vi "SA_Random_Solution.vi"(7 "Selection Method":T1, 8 "error in (no error)":errorcluster, 9 "Perturbation Method":T2=enum."NonRedundantSwap", 10 "GA.lvclass":refnum<class "GA.lvclass">, 11 "OSSP_Problem in":refnum<class "OSSP_Problem.lvclass">) -> (0 "error out":errorcluster, 2 "OSSP_Problem out":refnum<class "OSSP_Problem.lvclass">, 3 "GA out":refnum<class "GA.lvclass">)   [LabVIEW 2013]
uses:
  Classes/GA.lvclass
  Classes/OSSP_Problem.lvclass
  Classes/SA_Class/Controls/Perturbation Method.ctl
  Controls/SA Solution Selection Method.ctl
  Classes/SA.lvclass
  SA/Controls/States_SA.ctl
  Classes/OSSP_Problem.lvclass/OSSP_Problem.ctl
  Classes/GA.lvclass/GA.ctl
  Classes/SA_Class/Controls/CoolingScheme.ctl
  Classes/SA.lvclass/SA.ctl
  Classes/SA_Class/Controls/Solution_SA.ctl
  Classes/Graph.lvclass/Graph.ctl
  Classes/GA_Class/Controls/Solution_GA.ctl
  Classes/GanntChart_Class/Operation to Machine Job Tuple.vi
  Classes/GanntChart_Class/Check Other Machines for Schedule Time.vi
  Classes/GanntChart_Class/Schedule Job.vi
  Classes/GanntChart_Class/Find Gaps on Particular Machine.vi
  Classes/GanntChart_Class/Increment Number of Jobs on Machine.vi
  Classes/GanntChart_Class/Find Job On Other Machines.vi
  Remove Duplicates In Array.vi
  Classes/Graph_Class/Create Graph from Solution(Schedule).vi
  Classes/Graph_Class/Find All Paths_DFS.vi
  Classes/Graph_Class/Getters/Read Graph Dictionary.vi
  Classes/Graph_Class/Setters/Write Graph Dictionary.vi
  <userlib>/_OpenG.lib/array/array.llb/Filter 1D Array__ogtk.vi
  <userlib>/_OpenG.lib/array/array.llb/Filter 1D Array (I32)__ogtk.vi
  <userlib>/_OpenG.lib/array/array.llb/Remove Duplicates from 1D Array__ogtk.vi
  <userlib>/_OpenG.lib/array/array.llb/Remove Duplicates from 1D Array (I32)__ogtk.vi
  <userlib>/_OpenG.lib/array/array.llb/Search Array__ogtk.vi
  <userlib>/_OpenG.lib/array/array.llb/Search 1D Array (I32)__ogtk.vi
  <userlib>/_OpenG.lib/array/array.llb/Delete Elements from Array__ogtk.vi
  <userlib>/_OpenG.lib/array/array.llb/Delete Elements from 1D Array (I32)__ogtk.vi
  <userlib>/_OpenG.lib/array/array.llb/Sort Array__ogtk.vi
  <userlib>/_OpenG.lib/array/array.llb/Sort 1D Array (I32)__ogtk.vi
  <userlib>/_OpenG.lib/array/array.llb/Reorder Array2__ogtk.vi
  <userlib>/_OpenG.lib/array/array.llb/Reorder 1D Array2 (I32)__ogtk.vi
  Classes/Graph.lvclass
  Classes/GanntChart.lvclass
panel:
  out "Best Tardiness/Makespan":u16
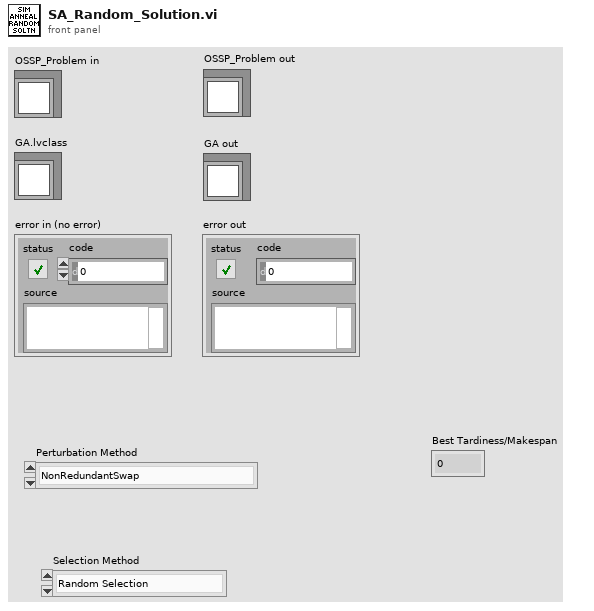
[diagram p1: front panel]
types:
  T1 = typedef "SA Solution Selection Method.ctl" = enum16{"Random Selection", "Tournament Selection"}
  T2 = typedef "SA.lvclass/Perturbation Method.ctl" = enum16{"Simple Swap", "Insert", "NonRedundantSwap", "Job Order Swap", "Machine Order Swap", "Machine&Job Order Swap", "Critical Path Swap"}
  T3 = typedef "States_SA.ctl" = enum16{"Init", "Read Problem", "Sort Problem", "Generate and Evaluate Current Solution", "Perturb Cur Solution and Eval New Solution", "Make Decision", "Keep Track of Best Solution", "Cool", "Output Final Solution", "Stop"}
  T4 = typedef "Solution_GA.ctl" = cluster{"Schedule":u16[], "Fitness":u16, "Fitness Valid?":bool}
  T5 = typedef "Scheduler Type.ctl" = enum16{"Non Delay Scheduler", "GT Active Scheduler", "FIFO Scheduler"}
  T6 = typedef "Objective.ctl" = enum16{"Makespan", "Total Tardiness"}
  T7 = typedef "SA.lvclass/CoolingScheme.ctl" = enum16{"Linear", "Geometric"}
  T8 = typedef "SA.lvclass/Solution_SA.ctl" = cluster{"Schedule":u16[], "Fitness":i16}
  T9 = typedef "GanntChart_Element.ctl" = cluster{"Operation Number":i32, "Job Number":i32, "Start Time":i32, "Procesing Time":u16, "End Time":i32}
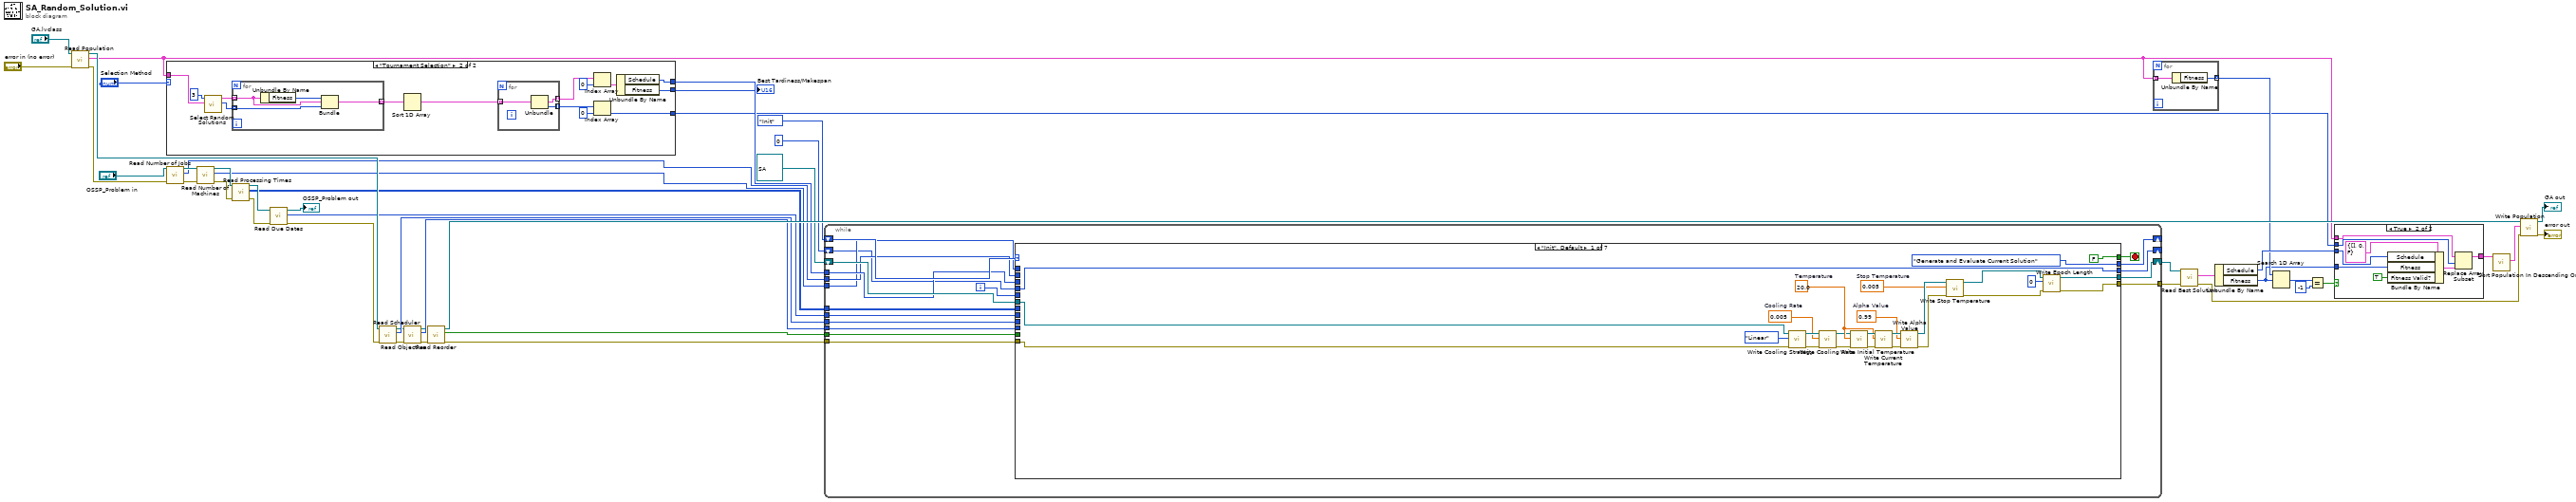
[diagram p0: block diagram]
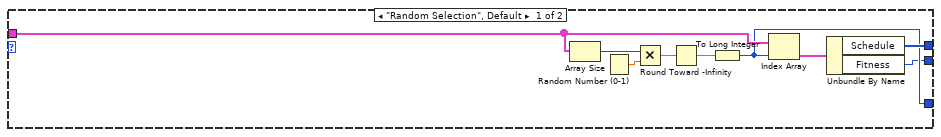
[diagram p2: hidden frame]
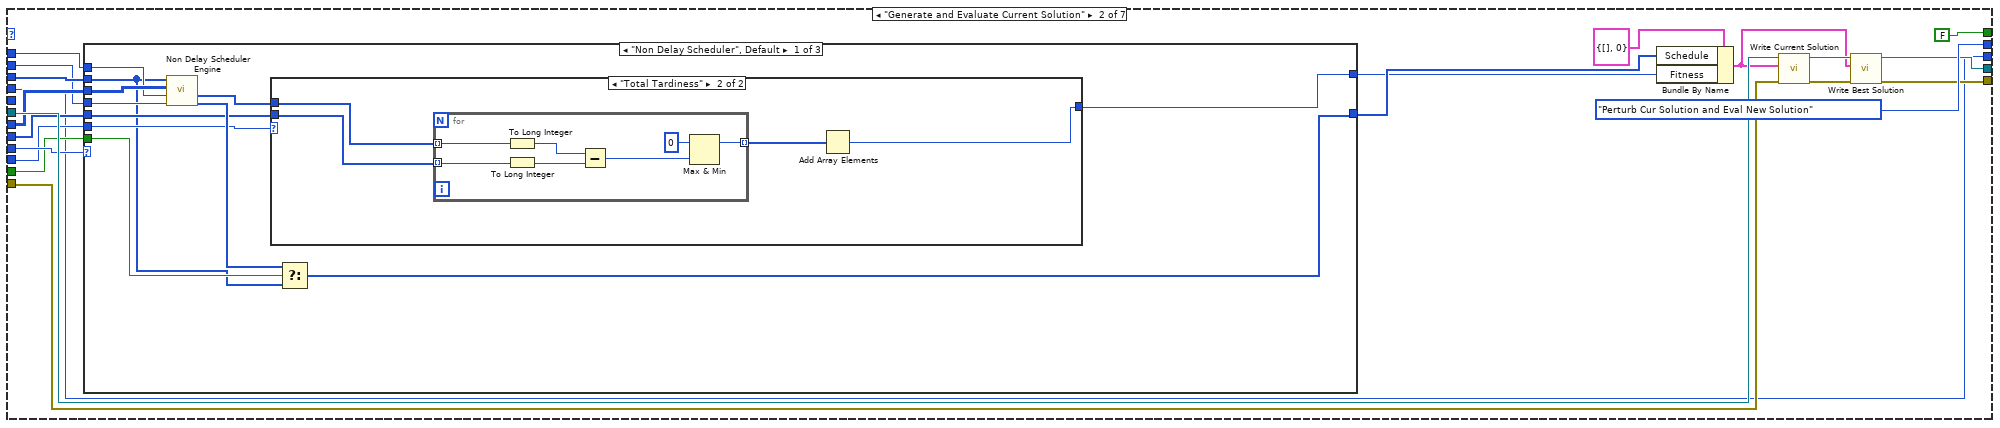
[diagram p4: hidden frame]
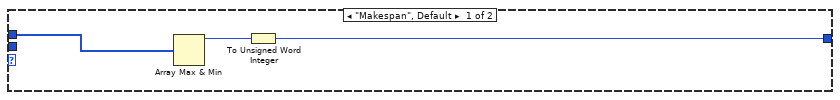
[diagram p5: hidden frame]
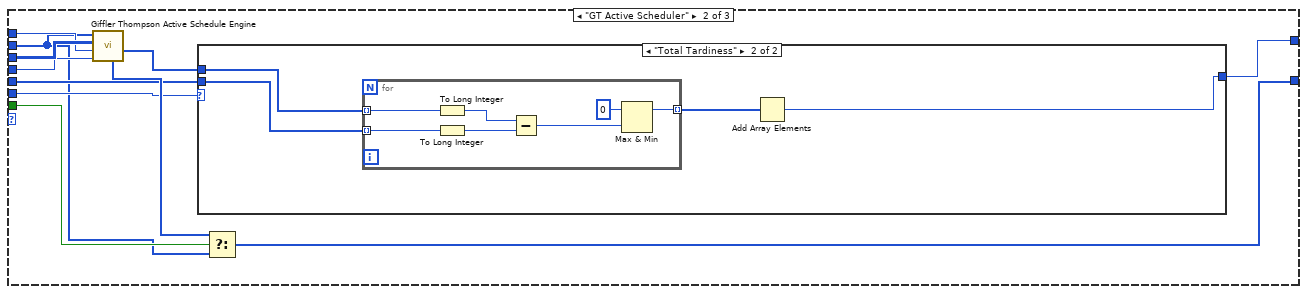
[diagram p6: hidden frame]
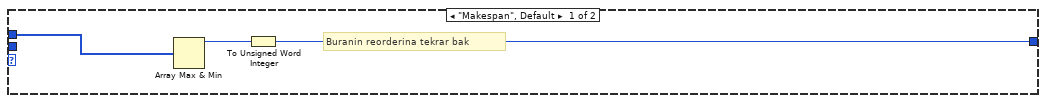
[diagram p7: hidden frame]
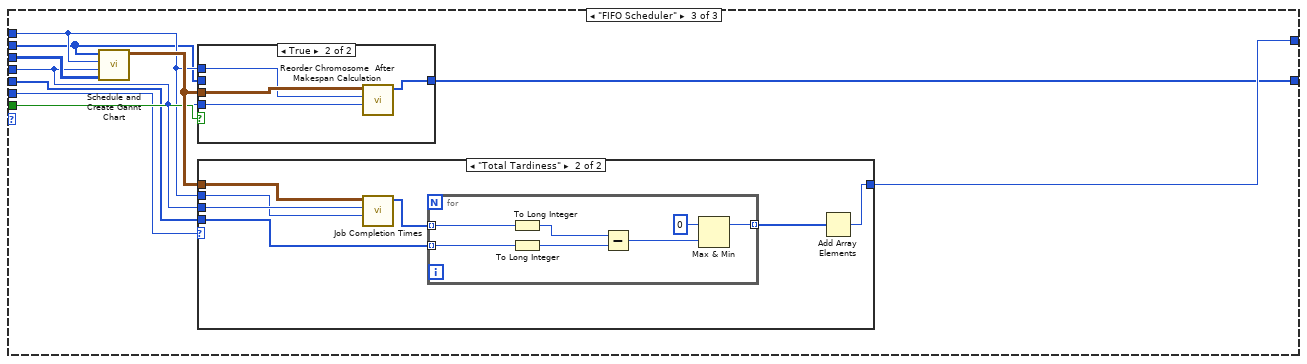
[diagram p8: hidden frame]
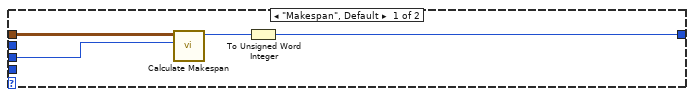
[diagram p10: hidden frame]
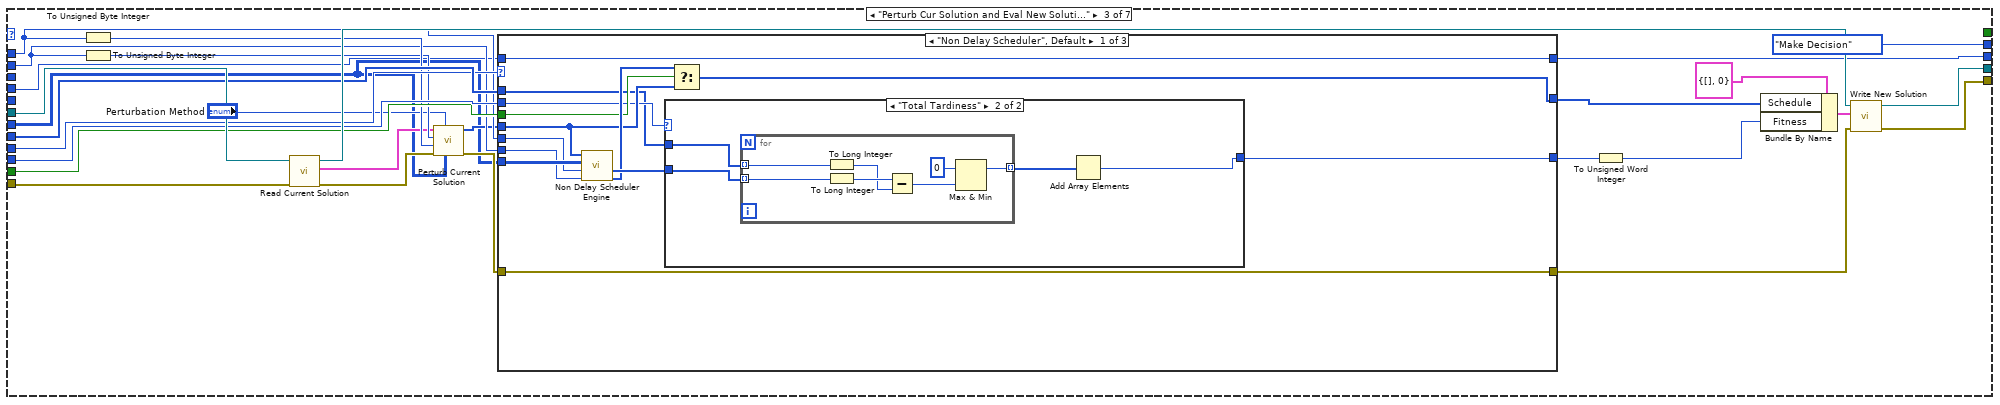
[diagram p11: hidden frame]
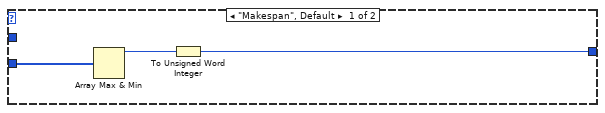
[diagram p12: hidden frame]
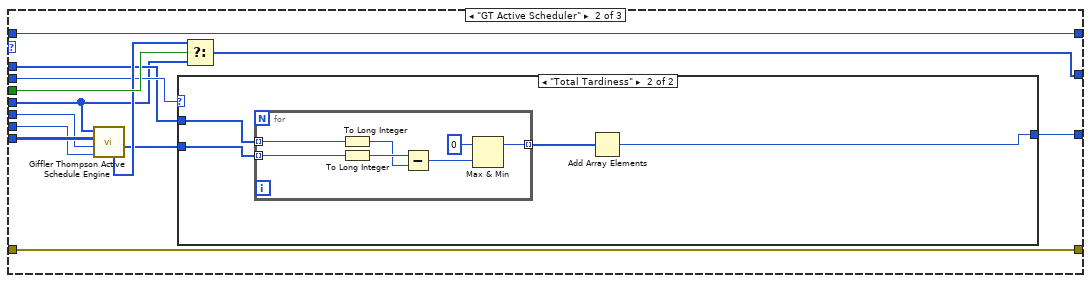
[diagram p13: hidden frame]
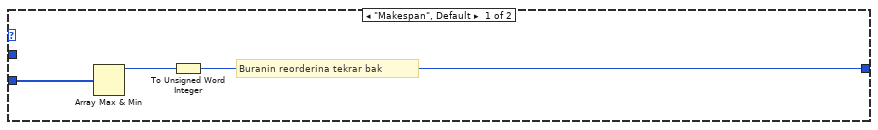
[diagram p14: hidden frame]
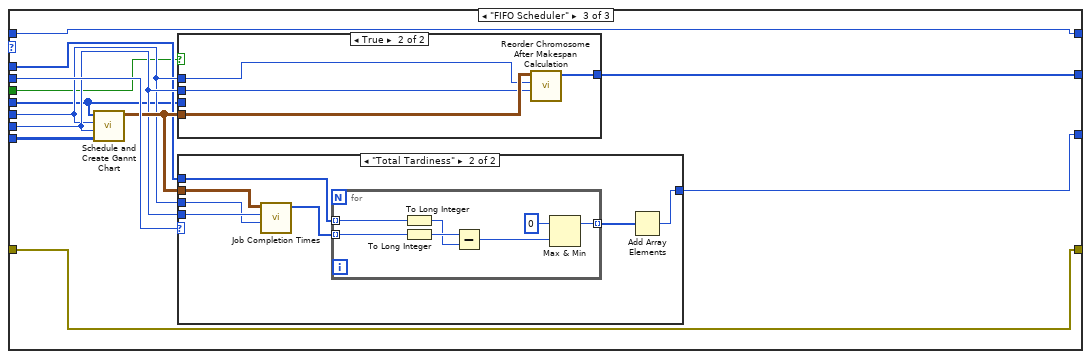
[diagram p15: hidden frame]
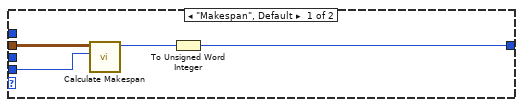
[diagram p17: hidden frame]
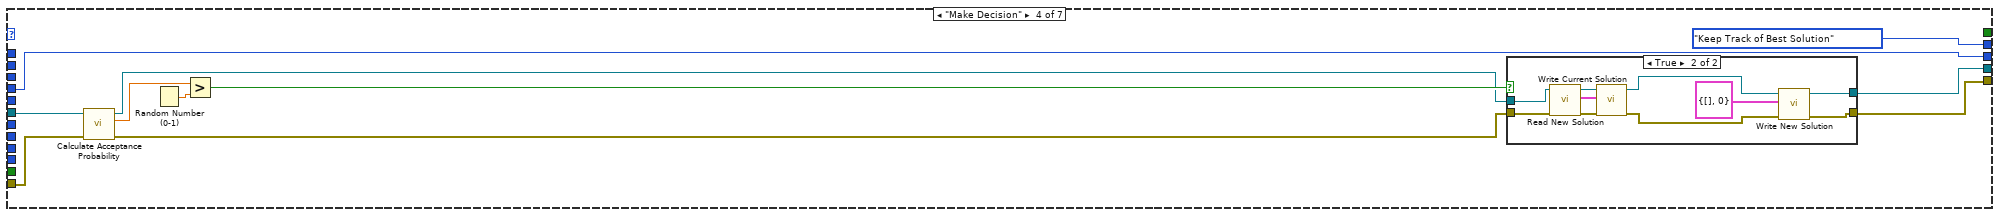
[diagram p18: hidden frame]
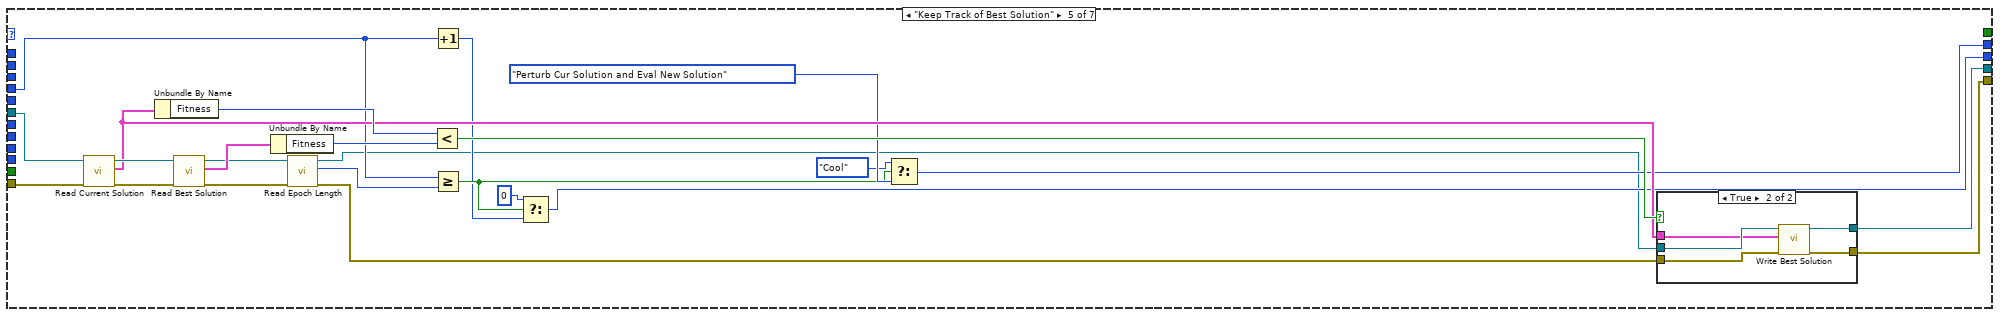
[diagram p20: hidden frame]
diagram:
  n1 = call-dynamic "Read Population.vi"("error in (no error)"="error in (no error)", "GA in"="GA.lvclass") -> ("error out"=w41:errorcluster, "Population"=w5:T4[], "GA out"=w42:refnum<class "GA.lvclass">)  [unwired: 7 in]
  n2 = case shown="\"Tournament Selection\"" "Selection Method" {
    tunnel: w5 -> [w53 w71]
    tunnel: [w51 w63] -> w4
    tunnel: [w50 w58] -> w3
    tunnel: [w49 w62] -> w2
    frame "Random Selection", Default {
      n3 = Array Size(array=w53) -> (size(s)=w56:i32)
      n4 = Random Number (0-1)() -> (number: 0 to 1=w57:dbl)
      n5 = Multiply(x=w56, y=w57) -> (x*y=w55:dbl)
      n6 = Round Toward -Infinity(1:w55) -> (0:w54:dbl)
      n7 = To Long Integer(number=w54) -> (32bit integer=w50:i32)
      n8 = Index Array(array=w53, index=w50) -> (element=w52:T4)
      n9 = Unbundle By Name(w52) -> ("Schedule"=w51:u16[], "Fitness"=w49:u16)
    }
    frame "Tournament Selection" {
      n10 = call "Select Random Solutions.vi"("Population"=w71, "Tournament Size"=3) -> ("Solution Indices"=w61:i32[], "Selected Solutions"=w69:T4[])  [unwired: 8 in]
      n11 = for {
        tunnel: w69 -> [w77] mode=indexing
        tunnel: [w76] -> w68 mode=indexing
        tunnel: w61 -> [w75] mode=indexing
        n12 = Unbundle By Name(w77) -> ("Fitness"=w78:u16)
        n13 = Bundle("Fitness"=w78, "Solution"=w77, w75) -> (w76:cluster{"Fitness":u16, "Solution":T4, i32})  [unwired: 1 in]
      }
      n14 = Sort 1D Array(array=w68) -> (sorted array=w65:cluster{"Fitness":u16, "Solution":T4, i32}[])
      n15 = for {
        tunnel: w65 -> [w74] mode=indexing
        tunnel: [w73] -> w67 mode=indexing
        tunnel: [w72] -> w60 mode=indexing
        n16 = Unbundle(w74) -> ("Solution"=w73:T4, w72:i32)  [unwired: 1 out]
      }
      n17 = Index Array(array=w67, index=0) -> (element=w64:T4)
      n18 = Index Array(array=w60, index=0) -> (element=w58:i32)
      n19 = Unbundle By Name(w64) -> ("Schedule"=w63:u16[], "Fitness"=w62:u16)
    }
  }
  "Best Tardiness/Makespan" <- w2
  n20 = call-dynamic "Read Number of Jobs.vi"("error in (no error)"=w41, "OSSP_Problem in"="OSSP_Problem in") -> ("error out"=w32:errorcluster, "Number of Jobs"=w36:i32, "OSSP_Problem out"=w38:refnum<class "OSSP_Problem.lvclass">)  [unwired: 7 in]
  n21 = call-dynamic "Read Number of Machines.vi"("error in (no error)"=w32, "OSSP_Problem in"=w38) -> ("error out"=w31:errorcluster, "Number of Machines"=w35:i32, "OSSP_Problem out"=w37:refnum<class "OSSP_Problem.lvclass">)  [unwired: 7 in]
  n22 = call-dynamic "Read Processing Times.vi"("error in (no error)"=w31, "OSSP_Problem in"=w37) -> ("error out"=w30:errorcluster, "Processing Times"=w14:u16[][], "OSSP_Problem out"=w29:refnum<class "OSSP_Problem.lvclass">)  [unwired: 7 in]
  n23 = call "Read Due Dates.vi"("error in (no error)"=w30, "OSSP_Problem in"=w29) -> ("error out"=w27:errorcluster, "Due Dates"=w28:u16[], "OSSP_Problem out"=→"OSSP_Problem out":refnum<class "OSSP_Problem.lvclass">)  [unwired: 7 in]
  n24 = call "Read Scheduler.vi"("error in (no error)"=w27, "GA in"=w42) -> ("error out"=w25:errorcluster, "Scheduler"=w26:T5, "GA out"=w24:refnum<class "GA.lvclass">)  [unwired: 7 in]
  n25 = call "Read Objective .vi"("error in (no error)"=w25, "GA in"=w24) -> ("error out"=w22:errorcluster, "Objective"=w23:T6, "GA out"=w19:refnum<class "GA.lvclass">)  [unwired: 7 in]
  n26 = call "Read Reorder.vi"("error in (no error)"=w22, "GA in"=w19) -> ("error out"=w21:errorcluster, "Reorder"=w20:bool, "GA out"=w43:refnum<class "GA.lvclass">)  [unwired: 7 in]
  n27 = while {
    tunnel: w4 -> [w94]
    shift-right: [w89] -> _
    shift-left: States_SA."Init" ("States") -> [w96]
    tunnel: w36 -> [w93]
    tunnel: w35 -> [w92]
    tunnel: w14 -> [w91]
    shift-right: [w90] -> w34
    shift-left: refnum<class "SA.lvclass"> refnum ("SA.lvclass") -> [w95]
    tunnel: [w87] -> w18
    tunnel: w21 -> [w86]
    tunnel: w28 -> [w85]
    tunnel: w26 -> [w84]
    tunnel: w23 -> [w83]
    tunnel: w20 -> [w82]
    shift-right: [w79] -> _
    shift-left: 0 -> [w80]
    i -> [w81]
    stop <- w88 stop-if-true
    n28 = case shown="\"Init\", Default" w96 {
      tunnel: w95 -> [w116 w142 w253 w353 w389 w402 w448]
      tunnel: w94 -> [_ w132 _ _ _ _ _]
      tunnel: w93 -> [_ w129 w236 _ _ _ _]
      tunnel: w92 -> [_ w130 w238 _ _ _ _]
      tunnel: w91 -> [_ w131 w228 _ _ _ _]
      tunnel: [w100 w137 w249 w352 w388 w407 w448] -> w90
      tunnel: [States_SA."Generate and Evaluate Current Solution" ("States") States_SA."Perturb Cur Solution and Eval New Solution" ("States") States_SA."Make Decision" ("States") States_SA."Keep Track of Best Solution" w376 w406 States_SA."Stop"] -> w89
      tunnel: [FALSE FALSE _ _ _ _ TRUE] -> w88
      tunnel: [w98 w123 w246 w345 w379 w404 w446] -> w87
      tunnel: w86 -> [w115 w124 w240 w347 w380 w400 w446]
      tunnel: w85 -> [_ w127 w243 _ _ _ _]
      tunnel: w84 -> [_ w135 w242 _ _ _ _]
      tunnel: w83 -> [_ w134 w241 _ _ _ _]
      tunnel: w82 -> [_ w133 w239 _ _ _ _]
      tunnel: w81 -> [_ _ _ _ _ w403 _]
      tunnel: w80 -> [w102 w122 w227 w344 w375 w397 w445]
      tunnel: [w102 w122 w226 w344 w371 w397 w445] -> w79
      frame "Init", Default {
        w108 = 0.005  # Stop Temperature
        w103 = 0.005  # Cooling Rate
        w120 = 0.99  # Alpha Value
        w111 = 20.0  # Temperature
        n29 = call "Write Cooling Strategy.vi"("error in (no error)"=w115, "Cooling Strategy"=CoolingScheme."Linear", "SA in"=w116) -> ("error out"=w105:errorcluster, "SA out"=w107:refnum<class "SA.lvclass">)  [unwired: 7 in]
        n30 = call "Write Cooling Rate.vi"("error in (no error)"=w105, "Cooling Rate"=w103, "SA in"=w107) -> ("error out"=w104:errorcluster, "SA out"=w106:refnum<class "SA.lvclass">)  [unwired: 7 in]
        n31 = call "Write Initial Temperature.vi"("error in (no error)"=w104, "Initial Temperature"=w111, "SA in"=w106) -> ("error out"=w112:errorcluster, "SA out"=w113:refnum<class "SA.lvclass">)  [unwired: 7 in]
        n32 = call "Write Current Temperature.vi"("error in (no error)"=w112, "Temperature"=w111, "SA in"=w113) -> ("error out"=w117:errorcluster, "SA out"=w121:refnum<class "SA.lvclass">)  [unwired: 7 in]
        n33 = call "Write Alpha Value.vi"("error in (no error)"=w117, "Alpha Value"=w120, "SA in"=w121) -> ("error out"=w109:errorcluster, "SA out"=w110:refnum<class "SA.lvclass">)  [unwired: 7 in]
        n34 = call "Write Stop Temperature.vi"("error in (no error)"=w109, "Stop Temperature"=w108, "SA in"=w110) -> ("error out"=w99:errorcluster, "SA out"=w101:refnum<class "SA.lvclass">)  [unwired: 7 in]
        n35 = call "Write Epoch Length.vi"("error in (no error)"=w99, "Epoch Length"=u8 0, "SA in"=w101) -> ("error out"=w98:errorcluster, "SA out"=w100:refnum<class "SA.lvclass">)  [unwired: 7 in]
      }
      frame "Generate and Evaluate Current Solution" {
        n36 = case shown="\"Non Delay Scheduler\", Default" w135 {
          tunnel: [w149 w174 w202] -> w126
          tunnel: [w150 w175 w200] -> w128
          tunnel: w132 -> [w143 w168 w193]
          tunnel: w133 -> [w151 w178 w199]
          tunnel: w134 -> [w148 w171 w196]
          tunnel: w131 -> [w147 w173 w198]
          tunnel: w130 -> [w146 w170 w195]
          tunnel: w129 -> [w145 w169 w194]
          tunnel: w127 -> [w144 w172 w197]
          frame "Non Delay Scheduler", Default {
            n37 = call "Non Delay Scheduler Engine.vi"("Number of  Jobs"=w145, "Number of Machines"=w146, "Processing Times"=w147, "Schedule"=w143) -> ("Scheduled Jobs Order"=w152:u16[], "Job Completion Times"=w153:u16[])  [unwired: 3 in, 3 out]
            n38 = case shown="\"Total Tardiness\"" w148 {
              tunnel: w153 -> [w156 w160]
              tunnel: [w154 w157] -> w149
              tunnel: w144 -> [_ w159]
              frame "Makespan", Default {
                n39 = Array Max & Min(array=w156) -> (max value=w155:u16)  [unwired: 3 out]
                n40 = To Unsigned Word Integer(number=w155) -> (unsigned 16bit integer=w154:u16)
              }
              frame "Total Tardiness" {
                n41 = for {
                  tunnel: w160 -> [w167] mode=indexing
                  tunnel: w159 -> [w166] mode=indexing
                  tunnel: [w161] -> w158 mode=indexing
                  n42 = To Long Integer(number=w167) -> (32bit integer=w165:i32)
                  n43 = To Long Integer(number=w166) -> (32bit integer=w164:i32)
                  n44 = Subtract(x=w165, y=w164) -> (x-y=w163:i32)
                  n45 = Max & Min(x=0, y=w163) -> (max(x,y)=w161:i32)  [unwired: 1 out]
                }
                n46 = Add Array Elements(numeric array=w158) -> (sum=w157:i32)
              }
            }
            n47 = Select(t=w152, s=w151, f=w143) -> (s? t:f=w150:u16[])
          }
          frame "GT Active Scheduler" {
            n48 = call "Giffler Thompson Active Schedule Engine.vi"("Number of  Jobs"=w169, "Number of Machines"=w170, "Processing Times"=w173, "Schedule In"=w168) -> ("Job Completion Times"=w176:u16[], "Schedule Order"=w177:u16[])  [unwired: 3 in, 3 out]
            n49 = case shown="\"Total Tardiness\"" w171 {
              tunnel: w176 -> [w181 w184]
              tunnel: [w179 w182] -> w174
              tunnel: w172 -> [_ w183]
              frame "Makespan", Default {
                # "Buranin reorderina tekrar bak"
                n50 = Array Max & Min(array=w181) -> (max value=w180:u16)  [unwired: 3 out]
                n51 = To Unsigned Word Integer(number=w180) -> (unsigned 16bit integer=w179:u16)
              }
              frame "Total Tardiness" {
                n52 = for {
                  tunnel: [w188] -> w185 mode=indexing
                  tunnel: w184 -> [w187] mode=indexing
                  tunnel: w183 -> [w186] mode=indexing
                  n53 = To Long Integer(number=w187) -> (32bit integer=w192:i32)
                  n54 = To Long Integer(number=w186) -> (32bit integer=w191:i32)
                  n55 = Subtract(x=w192, y=w191) -> (x-y=w190:i32)
                  n56 = Max & Min(x=0, y=w190) -> (max(x,y)=w188:i32)  [unwired: 1 out]
                }
                n57 = Add Array Elements(numeric array=w185) -> (sum=w182:i32)
              }
            }
            n58 = Select(t=w177, s=w178, f=w168) -> (s? t:f=w175:u16[])
          }
          frame "FIFO Scheduler" {
            n59 = call "Schedule and Create Gannt Chart.vi"("Processing Times (Rows Mach.Cols Jobs)"=w198, "Number of Jobs"=w194, "Number of Machines"=w195, "Schedule"=w193) -> ("Gannt Chart Out"=w201:T9[][])  [unwired: 6 in, 1 out]
            n60 = case shown="True" w199 {
              tunnel: w201 -> [_ w207]
              tunnel: [w203 w206] -> w200
              tunnel: w195 -> [_ w205]
              tunnel: w194 -> [_ w204]
              tunnel: w193 -> [w203 _]
              frame False {
              }
              frame True {
                n61 = call "Reorder Chromosome  After Makespan Calculation.vi"("Number Of  Jobs"=w204, "Number Of Machines"=w205, "Gannt Chart In"=w207) -> ("Reordered Chromosome"=w206:u16[])  [unwired: 8 in]
              }
            }
            n62 = case shown="\"Total Tardiness\"" w196 {
              tunnel: w201 -> [w211 w218]
              tunnel: [w209 w212] -> w202
              tunnel: w197 -> [_ w213]
              tunnel: w194 -> [w208 w217]
              tunnel: w195 -> [_ w216]
              frame "Makespan", Default {
                n63 = call "Calculate Makespan.vi"("Number of Jobs"=w208, "Gannt Chart In"=w211) -> ("Makespan"=w210:i32)  [unwired: 9 in]
                n64 = To Unsigned Word Integer(number=w210) -> (unsigned 16bit integer=w209:u16)
              }
              frame "Total Tardiness" {
                n65 = call "Job Completion Times.vi"("Number Of Machines"=w216, "Number Of Jobs"=w217, "Gannt Chart In"=w218) -> ("Job Completion Times"=w214:u16[])  [unwired: 8 in]
                n66 = for {
                  tunnel: [w221] -> w215 mode=indexing
                  tunnel: w214 -> [w220] mode=indexing
                  tunnel: w213 -> [w219] mode=indexing
                  n67 = To Long Integer(number=w220) -> (32bit integer=w225:i32)
                  n68 = To Long Integer(number=w219) -> (32bit integer=w224:i32)
                  n69 = Subtract(x=w225, y=w224) -> (x-y=w223:i32)
                  n70 = Max & Min(x=0, y=w223) -> (max(x,y)=w221:i32)  [unwired: 1 out]
                }
                n71 = Add Array Elements(numeric array=w215) -> (sum=w212:i32)
              }
            }
          }
        }
        n72 = Bundle By Name(cluster=T8 {"Schedule"=[], "Fitness"=0} ("Solution"), "Schedule"=w128, "Fitness"=w126) -> (w136:T8)
        n73 = call "Write Current Solution.vi"("error in (no error)"=w124, "Solution"=w136, "SA in"=w142) -> ("error out"=w125:errorcluster, "SA out"=w138:refnum<class "SA.lvclass">)  [unwired: 7 in]
        n74 = call "Write Best Solution.vi"("error in (no error)"=w125, "Solution"=w136, "SA in"=w138) -> ("error out"=w123:errorcluster, "SA out"=w137:refnum<class "SA.lvclass">)  [unwired: 7 in]
      }
      frame "Perturb Cur Solution and Eval New Solution" {
        n75 = To Unsigned Byte Integer(number=w238) -> (unsigned 8bit integer=w237:u8)
        n76 = To Unsigned Byte Integer(number=w236) -> (unsigned 8bit integer=w235:u8)
        n77 = call "Read Current Solution.vi"("error in (no error)"=w240, "SA in"=w253) -> ("error out"=w233:errorcluster, "Solution"=w229:T8, "SA out"=w252:refnum<class "SA.lvclass">)  [unwired: 7 in]
        n78 = call "Perturb Current Solution.vi"("Processing Times (Rows Machine, Columns Jobs)"=w228, "Perturbation Method"="Perturbation Method", "error in (no error)"=w233, "Number of Machines"=w237, "Number of Jobs"=w235, "Solution"=w229) -> ("error out"=w232:errorcluster, "Perturbed Schedule"=w230:u16[])  [unwired: 4 in]
        n79 = case shown="\"Non Delay Scheduler\", Default" w242 {
          tunnel: w230 -> [w260 w285 w310]
          tunnel: w238 -> [w262 w287 w313]
          tunnel: w236 -> [w263 w289 w315]
          tunnel: w228 -> [w264 w293 w319]
          tunnel: [w256 w283 w318] -> w245
          tunnel: w241 -> [w258 w288 w317]
          tunnel: [w259 w284 w314] -> w244
          tunnel: w243 -> [w257 w286 w312]
          tunnel: w239 -> [w261 w292 w311]
          tunnel: [w255 w282 w309] -> w231
          tunnel: w232 -> [w255 w282 w309]
          tunnel: w227 -> [w254 w281 w308]
          tunnel: [w254 w281 w308] -> w226
          frame "Non Delay Scheduler", Default {
            n80 = call "Non Delay Scheduler Engine.vi"("Number of  Jobs"=w263, "Number of Machines"=w262, "Processing Times"=w264, "Schedule"=w260) -> ("Scheduled Jobs Order"=w265:u16[], "Job Completion Times"=w266:u16[])  [unwired: 3 in, 3 out]
            n81 = case shown="\"Total Tardiness\"" w258 {
              tunnel: w266 -> [w269 w272]
              tunnel: [w267 w270] -> w256
              tunnel: w257 -> [_ w271]
              frame "Makespan", Default {
                n82 = Array Max & Min(array=w269) -> (max value=w268:u16)  [unwired: 3 out]
                n83 = To Unsigned Word Integer(number=w268) -> (unsigned 16bit integer=w267:u16)
              }
              frame "Total Tardiness" {
                n84 = for {
                  tunnel: w272 -> [w280] mode=indexing
                  tunnel: w271 -> [w279] mode=indexing
                  tunnel: [w274] -> w273 mode=indexing
                  n85 = To Long Integer(number=w279) -> (32bit integer=w277:i32)
                  n86 = To Long Integer(number=w280) -> (32bit integer=w278:i32)
                  n87 = Subtract(x=w278, y=w277) -> (x-y=w276:i32)
                  n88 = Max & Min(x=0, y=w276) -> (max(x,y)=w274:i32)  [unwired: 1 out]
                }
                n89 = Add Array Elements(numeric array=w273) -> (sum=w270:i32)
              }
            }
            n90 = Select(t=w265, s=w261, f=w260) -> (s? t:f=w259:u16[])
          }
          frame "GT Active Scheduler" {
            n91 = call "Giffler Thompson Active Schedule Engine.vi"("Number of  Jobs"=w289, "Number of Machines"=w287, "Processing Times"=w293, "Schedule In"=w285) -> ("Job Completion Times"=w290:u16[], "Schedule Order"=w291:u16[])  [unwired: 3 in, 3 out]
            n92 = case shown="\"Total Tardiness\"" w288 {
              tunnel: w290 -> [w296 w299]
              tunnel: [w294 w297] -> w283
              tunnel: w286 -> [_ w298]
              frame "Makespan", Default {
                # "Buranin reorderina tekrar bak"
                n93 = Array Max & Min(array=w296) -> (max value=w295:u16)  [unwired: 3 out]
                n94 = To Unsigned Word Integer(number=w295) -> (unsigned 16bit integer=w294:u16)
              }
              frame "Total Tardiness" {
                n95 = for {
                  tunnel: [w303] -> w300 mode=indexing
                  tunnel: w299 -> [w302] mode=indexing
                  tunnel: w298 -> [w301] mode=indexing
                  n96 = To Long Integer(number=w301) -> (32bit integer=w306:i32)
                  n97 = To Long Integer(number=w302) -> (32bit integer=w307:i32)
                  n98 = Subtract(x=w307, y=w306) -> (x-y=w305:i32)
                  n99 = Max & Min(x=0, y=w305) -> (max(x,y)=w303:i32)  [unwired: 1 out]
                }
                n100 = Add Array Elements(numeric array=w300) -> (sum=w297:i32)
              }
            }
            n101 = Select(t=w291, s=w292, f=w285) -> (s? t:f=w284:u16[])
          }
          frame "FIFO Scheduler" {
            n102 = call "Schedule and Create Gannt Chart.vi"("Processing Times (Rows Mach.Cols Jobs)"=w319, "Number of Jobs"=w315, "Number of Machines"=w313, "Schedule"=w310) -> ("Gannt Chart Out"=w316:T9[][])  [unwired: 6 in, 1 out]
            n103 = case shown="True" w311 {
              tunnel: w316 -> [_ w324]
              tunnel: w313 -> [_ w323]
              tunnel: w315 -> [_ w322]
              tunnel: [w320 w321] -> w314
              tunnel: w310 -> [w320 _]
              frame False {
              }
              frame True {
                n104 = call "Reorder Chromosome  After Makespan Calculation.vi"("Number Of  Jobs"=w322, "Number Of Machines"=w323, "Gannt Chart In"=w324) -> ("Reordered Chromosome"=w321:u16[])  [unwired: 8 in]
              }
            }
            n105 = case shown="\"Total Tardiness\"" w317 {
              tunnel: w316 -> [w328 w335]
              tunnel: [w325 w329] -> w318
              tunnel: w315 -> [w327 w334]
              tunnel: w313 -> [_ w333]
              tunnel: w312 -> [_ w330]
              frame "Makespan", Default {
                n106 = call "Calculate Makespan.vi"("Number of Jobs"=w327, "Gannt Chart In"=w328) -> ("Makespan"=w326:i32)  [unwired: 9 in]
                n107 = To Unsigned Word Integer(number=w326) -> (unsigned 16bit integer=w325:u16)
              }
              frame "Total Tardiness" {
                n108 = call "Job Completion Times.vi"("Number Of Machines"=w333, "Number Of Jobs"=w334, "Gannt Chart In"=w335) -> ("Job Completion Times"=w331:u16[])  [unwired: 8 in]
                n109 = for {
                  tunnel: [w338] -> w332 mode=indexing
                  tunnel: w331 -> [w337] mode=indexing
                  tunnel: w330 -> [w336] mode=indexing
                  n110 = To Long Integer(number=w336) -> (32bit integer=w341:i32)
                  n111 = To Long Integer(number=w337) -> (32bit integer=w342:i32)
                  n112 = Subtract(x=w342, y=w341) -> (x-y=w340:i32)
                  n113 = Max & Min(x=0, y=w340) -> (max(x,y)=w338:i32)  [unwired: 1 out]
                }
                n114 = Add Array Elements(numeric array=w332) -> (sum=w329:i32)
              }
            }
          }
        }
        n115 = To Unsigned Word Integer(number=w245) -> (unsigned 16bit integer=w247:u16)
        n116 = Bundle By Name(cluster=T8 {"Schedule"=[], "Fitness"=0} ("Solution"), "Schedule"=w244, "Fitness"=w247) -> (w250:T8)
        n117 = call "Write New Solution.vi"("error in (no error)"=w231, "Solution"=w250, "SA in"=w252) -> ("error out"=w246:errorcluster, "SA out"=w249:refnum<class "SA.lvclass">)  [unwired: 7 in]
      }
      frame "Make Decision" {
        n118 = call "Calculate Acceptance Probability.vi"("error in (no error)"=w347, "SA in"=w353) -> ("error out"=w346:errorcluster, "Acceptance Probability"=w351:dbl, "SA out"=w348:refnum<class "SA.lvclass">)  [unwired: 7 in]
        n119 = Random Number (0-1)() -> (number: 0 to 1=w350:dbl)
        n120 = Greater?(x=w351, y=w350) -> (0:w349:bool)
        n121 = case shown="True" w349 {
          tunnel: w348 -> [w355 w365]
          tunnel: [w355 w359] -> w352
          tunnel: w346 -> [w354 w358]
          tunnel: [w354 w357] -> w345
          frame False {
          }
          frame True {
            n122 = call "Read New Solution.vi"("error in (no error)"=w358, "SA in"=w365) -> ("error out"=w364:errorcluster, "Solution"=w362:T8, "SA out"=w363:refnum<class "SA.lvclass">)  [unwired: 7 in]
            n123 = call "Write Current Solution.vi"("error in (no error)"=w364, "Solution"=w362, "SA in"=w363) -> ("error out"=w360:errorcluster, "SA out"=w361:refnum<class "SA.lvclass">)  [unwired: 7 in]
            n124 = call "Write New Solution.vi"("error in (no error)"=w360, "Solution"=T8 {"Schedule"=[], "Fitness"=0}, "SA in"=w361) -> ("error out"=w357:errorcluster, "SA out"=w359:refnum<class "SA.lvclass">)  [unwired: 7 in]
          }
        }
      }
      frame "Keep Track of Best Solution" {
        n125 = call "Read Current Solution.vi"("error in (no error)"=w380, "SA in"=w389) -> ("error out"=w381:errorcluster, "Solution"=w382:T8, "SA out"=w387:refnum<class "SA.lvclass">)  [unwired: 7 in]
        n126 = Unbundle By Name(w382) -> ("Fitness"=w386:i16)
        n127 = call "Read Best Solution.vi"("error in (no error)"=w381, "SA in"=w387) -> ("error out"=w367:errorcluster, "Solution"=w385:T8, "SA out"=w370:refnum<class "SA.lvclass">)  [unwired: 7 in]
        n128 = Unbundle By Name(w385) -> ("Fitness"=w384:i16)
        n129 = call "Read Epoch Length.vi"("error in (no error)"=w367, "SA in"=w370) -> ("error out"=w366:errorcluster, "Epoch Length"=w368:u8, "SA out"=w369:refnum<class "SA.lvclass">)  [unwired: 7 in]
        n130 = Less?(x=w386, y=w384) -> (x < y?=w383:bool)
        n131 = Increment(x=w375) -> (x+1=w373:i32)
        n132 = Greater Or Equal?(x=w375, y=w368) -> (x >= y?=w374:bool)
        n133 = Select(t=0, s=w374, f=w373) -> (s? t:f=w371:i32)
        n134 = Select(t=States_SA."Cool", s=w374, f=States_SA."Perturb Cur Solution and Eval New Solution") -> (s? t:f=w376:T3)
        n135 = case shown="True" w383 {
          tunnel: w369 -> [w391 w396]
          tunnel: [w391 w395] -> w388
          tunnel: w382 -> [_ w394]
          tunnel: w366 -> [w390 w393]
          tunnel: [w390 w392] -> w379
          frame False {
          }
          frame True {
            n136 = call "Write Best Solution.vi"("error in (no error)"=w393, "Solution"=w394, "SA in"=w396) -> ("error out"=w392:errorcluster, "SA out"=w395:refnum<class "SA.lvclass">)  [unwired: 7 in]
          }
        }
      }
      frame "Cool" {
        n137 = call "Read Stop Temperature.vi"("error in (no error)"=w400, "SA in"=w402) -> ("error out"=w399:errorcluster, "Stop Temperature"=w398:dbl, "SA out"=w401:refnum<class "SA.lvclass">)  [unwired: 7 in]
        n138 = call "Read Current Temperature.vi"("error in (no error)"=w399, "SA in"=w401) -> ("error out"=w405:errorcluster, "Temperature"=w408:dbl, "SA out"=w409:refnum<class "SA.lvclass">)  [unwired: 7 in]
        n139 = Less?(x=w408, y=w398) -> (x < y?=w410:bool)
        n140 = case shown="False" w410 {
          tunnel: [States_SA."Perturb Cur Solution and Eval New Solution" ("f") States_SA."Stop"] -> w406
          tunnel: w409 -> [w416 w443]
          tunnel: [w422 w443] -> w407
          tunnel: w408 -> [w418 _]
          tunnel: w405 -> [w414 w442]
          tunnel: [w417 w442] -> w404
          tunnel: w403 -> [w411 _]
          frame False {
            n141 = call "Read Cooling Strategy.vi"("error in (no error)"=w414, "SA in"=w416) -> ("error out"=w413:errorcluster, "Cooling Strategy"=w412:T7, "SA out"=w415:refnum<class "SA.lvclass">)  [unwired: 7 in]
            n142 = case shown="\"Geometric\"" w412 {
              tunnel: w415 -> [w432 w441]
              tunnel: [w431 w433] -> w421
              tunnel: [w430 w436] -> w420
              tunnel: [w426 w439] -> w419
              tunnel: w418 -> [w425 _]
              tunnel: w413 -> [w424 w440]
              tunnel: w411 -> [_ _]
              frame "Linear", Default {
                n143 = call "Read Cooling Rate.vi"("error in (no error)"=w424, "SA in"=w432) -> ("error out"=w430:errorcluster, "Cooling Rate"=w428:dbl, "SA out"=w431:refnum<class "SA.lvclass">)  [unwired: 7 in]
                n144 = Subtract(x=1.0, y=w428) -> (x-y=w427:dbl)
                n145 = Multiply(x=w427, y=w425) -> (x*y=w426:dbl)
              }
              frame "Geometric" {
                n146 = call "Read Alpha Value.vi"("error in (no error)"=w440, "SA in"=w441) -> ("error out"=w437:errorcluster, "Alpha Value"=w435:dbl, "SA out"=w438:refnum<class "SA.lvclass">)  [unwired: 7 in]
                n147 = call "Read Current Temperature.vi"("error in (no error)"=w437, "SA in"=w438) -> ("error out"=w436:errorcluster, "Temperature"=w434:dbl, "SA out"=w433:refnum<class "SA.lvclass">)  [unwired: 7 in]
                n148 = Multiply(x=w435, y=w434) -> (x*y=w439:dbl)
              }
            }
            n149 = call "Write Current Temperature.vi"("error in (no error)"=w420, "Temperature"=w419, "SA in"=w421) -> ("error out"=w417:errorcluster, "SA out"=w422:refnum<class "SA.lvclass">)  [unwired: 7 in]
          }
          frame True {
          }
        }
      }
      frame "Stop" {
      }
    }
  }
  n150 = for {
    tunnel: w5 -> [w451] mode=indexing
    tunnel: [w450] -> w10 mode=indexing
    n151 = Unbundle By Name(w451) -> ("Fitness"=w450:u16)
  }
  n152 = call "Read Best Solution.vi"("error in (no error)"=w18, "SA in"=w34) -> ("error out"=w17:errorcluster, "Solution"=w33:T8)  [unwired: 7 in, 1 out]
  n153 = Unbundle By Name(w33) -> ("Schedule"=w15:u16[], "Fitness"=w9:i16)
  n154 = Search 1D Array(1D array=w10, element=w9) -> (index of element=w12:i32)  [unwired: 1 in]
  n155 = Equal?(x=w12, y=-1) -> (x = y?=w8:bool)
  n156 = case shown="True" w8 {
    tunnel: [w452 w459] -> w7
    tunnel: w15 -> [_ w456]
    tunnel: w3 -> [_ w455]
    tunnel: w5 -> [w452 w454]
    tunnel: w9 -> [_ w453]
    frame False {
    }
    frame True {
      n157 = Bundle By Name(cluster=T4 {"Schedule"=[], "Fitness"=0, "Fitness Valid?"=FALSE} ("new element/subarray"), "Schedule"=w456, "Fitness"=w453, "Fitness Valid?"=TRUE) -> (w460:T4)
      n158 = Replace Array Subset(array=w454, new element=w460, index=w455) -> (w459:T4[])
    }
  }
  n159 = call "Sort Population In Descending Order.vi"("Population"=w7) -> ("Population In Descending Order"=w6:T4[])  [unwired: 9 in, 1 out]
  n160 = call "Write Population.vi"("error in (no error)"=w17, "Population"=w6, "GA in"=w43) -> ("error out"=→"error out":errorcluster, "GA out"=→"GA out":refnum<class "GA.lvclass">)  [unwired: 7 in]
